vi "DAQNavi Write (Digital 2D U8 NChan NSamp).vi"(8 "error in (no error)":errorcluster, 9 "timeout":dbl=10.0, 10 "data":u8[][](array[numeric]), 11 "task in":i32) -> (0 "error out":errorcluster, 2 "number of samples written per channel":u32, 3 "task out":i32)   [LabVIEW 2020]
uses:
  DAQNavi_LV.dll
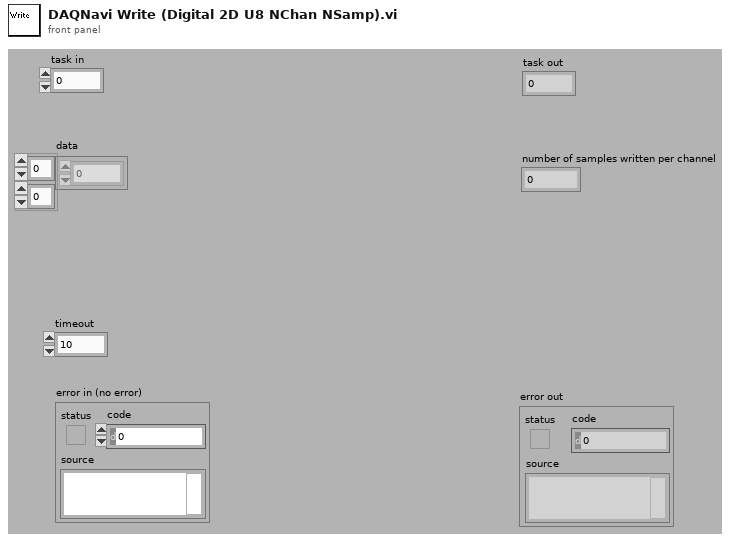
[diagram p1: front panel]
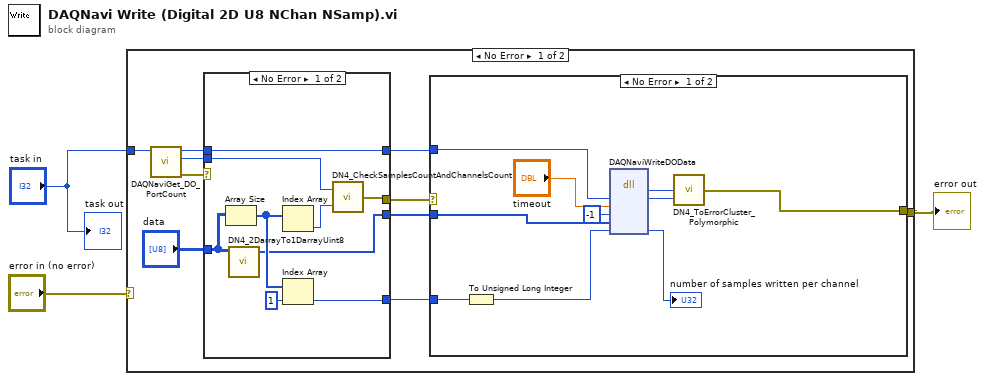
[diagram p0: block diagram]
diagram:
  n1 = case shown="No Error" "error in (no error)" {
    selector: "error in (no error)" -> [_ w36]
    tunnel: [w9 w36] -> w2
    tunnel: "task in" -> [w10 _]
    frame No Error {
      n2 = call "DAQNaviGet_DO_PortCount.vi"("task in"=w10) -> ("error out"=w13:errorcluster, "port count"=w12:i32, "task out"=w11:i32)  [unwired: 1 in, 7 out]
      n3 = case shown="No Error" w13 {
        selector: w13 -> [_ w24]
        tunnel: w12 -> [w21 _]
        tunnel: [w20 w24] -> w7
        tunnel: [w22 w23] -> w8
        tunnel: w11 -> [w22 w23]
        tunnel: "data" -> [w15 _]
        tunnel: [w14 _] -> w5
        tunnel: [w16 _] -> w4
        frame No Error {
          n4 = Array Size(array=w15) -> (size(s)=w18:i32[])
          n5 = call "DN4_2DarrayTo1DarrayUint8.vi"("2Darray"=w15) -> ("1Darray"=w14:u8[])  [unwired: 5 out]
          n6 = Index Array(array=w18) -> (element=w19:i32)  [unwired: 1 in]
          n7 = Index Array(array=w18, index=1) -> (element=w16:i32)
          n8 = call "DN4_CheckSamplesCountAndChannelsCount.vi"("samples count"=w19, "channel count"=w21) -> ("error out"=w20:errorcluster)
        }
        frame Error {
        }
      }
      n9 = case shown="No Error" w7 {
        selector: w7 -> [_ w35]
        tunnel: [w34 w35] -> w9
        tunnel: w8 -> [w30 _]
        tunnel: w5 -> [w27 _]
        tunnel: w4 -> [w29 _]
        frame No Error {
          n10 = To Unsigned Long Integer(number=w29) -> (unsigned 32bit integer=w28:u32)
          n11 = dll-call lib="DAQNavi_LV.dll" fn="DAQNaviWriteDOData"("taskID"=w30, "timeout"="timeout", "portBit"=-1, "portData"=w27, "samples"=w28) -> ("return type"=w31:i32, "taskID"=w26:i32, "samples"=→"number of samples written per channel":u32)  [unwired: 6 in, 2 out]
          n12 = call "DN4_ToErrorCluster_Polymorphic.vi"("task id"=w26, "error code"=w31) -> ("error out"=w34:errorcluster)  [unwired: 3 out]
        }
        frame Error {
        }
      }
    }
    frame Error {
    }
  }
  "error out" <- w2
  "task out" <- "task in"
